vi "Open VI Flag Generation.vi"(10 "Call And Collect (F)":bool, 11 "Re-entrant (F)":bool) -> (3 "Flags":i32 format="%.0x")   [LabVIEW 2015, in "Actor.lvclass"]
uses:
  Actor.lvclass
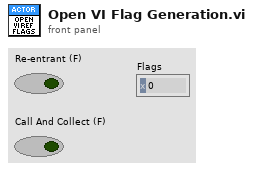
[diagram p1: front panel]
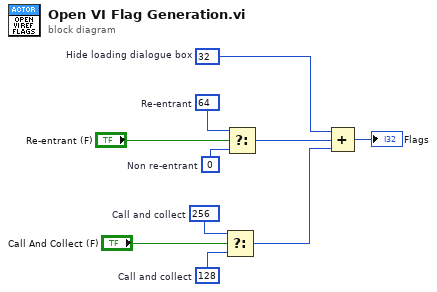
[diagram p0: block diagram]
diagram:
  w3 = 0  # Non re-entrant
  w2 = 64  # Re-entrant
  w6 = 128  # Call and collect
  w7 = 256  # Call and collect
  w9 = 32  # Hide loading dialogue box
  n1 = Select(t=w7, s="Call And Collect (F)", f=w6) -> (s? t:f=w5:i32)
  n2 = Select(t=w2, s="Re-entrant (F)", f=w3) -> (s? t:f=w1:i32)
  n3 = Compound Arithmetic op=ADD(w9, w1, w5) -> (→"Flags":i32)
